vi "Get Start and End Time.vi"(2 "Binary Data":u8[](array[numeric])) -> (7 "Start Time":dbl, 9 "End Time":dbl)   [LabVIEW 2020]
panel:
  out "Binary Data 2":u8[](array[numeric])
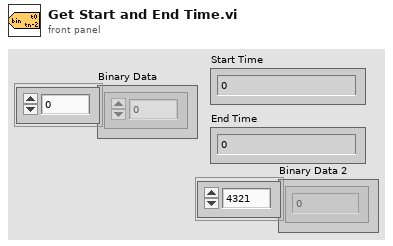
[diagram p1: front panel]
types:
  T1 = typedef "gyro_control_measurement_settings.ctl" = cluster{"# Pages":i32, "ODR":u8, "xlRange":u8, "gyroRange":u8, "id":u8, "Samplig Freq [Hz]":dbl, "xlRange in g":dbl, "gyroRange in dps":dbl}
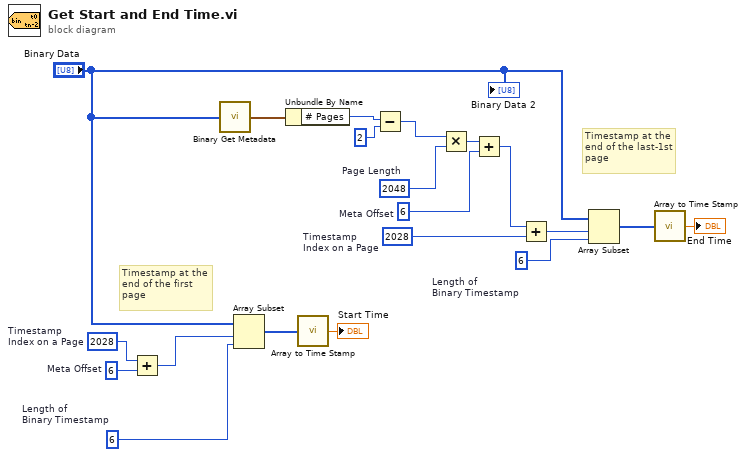
[diagram p0: block diagram]
diagram:
  w8 = 2028  # Timestamp Index on a Page
  w10 = 6  # Meta Offset
  w12 = 6  # Length of  Binary Timestamp
  w16 = 6  # Length of  Binary Timestamp
  w14 = 2048  # Page Length
  w18 = 6  # Meta Offset
  w19 = 2028  # Timestamp Index on a Page
  # "Timestamp at the end of the last-1st page"
  # "Timestamp at the end of the first page"
  n1 = Add(x=w19, y=w18) -> (x+y=w17:i32)
  n2 = call "Binary Get Metadata.vi"("Binary Data"="Binary Data") -> ("Meta"=w4:T1)  [unwired: 4 in]
  n3 = Array Subset(array="Binary Data", index=w17, length=w16) -> (w6:u8[])
  n4 = Unbundle By Name(w4) -> ("# Pages"=w1:i32)
  n5 = call "Array to Time Stamp.vi"("6 Byte Times Stamp"=w6) -> ("Seconds as DBL"=→"Start Time":dbl)  [unwired: 13 in, 1 out]
  n6 = Subtract(x=w1, y=2) -> (x-y=w20:i32)
  n7 = Multiply(x=w20, y=w14) -> (x*y=w11:i32)
  n8 = Add(x=w11, y=w10) -> (x+y=w9:i32)
  n9 = Add(x=w9, y=w8) -> (x+y=w7:i32)
  n10 = Array Subset(array="Binary Data", index=w7, length=w12) -> (w5:u8[])
  n11 = call "Array to Time Stamp.vi"("6 Byte Times Stamp"=w5) -> ("Seconds as DBL"=→"End Time":dbl)  [unwired: 13 in, 1 out]
  "Binary Data 2" <- "Binary Data"
